vi "zad3 v0.0.2.vi"() -> ()   [LabVIEW 2017]
panel:
  in  "Interval (ms)":u32=500
  in  "stop":bool
  out "AIN3":dbl format="%.6f"
  out "AIN2":dbl format="%.6f"
  in  "FIO7":bool
  in  "FIO6":bool
  in  "DAC0":dbl format="%.4f"
  out "Error Message":string
  out "error out":errorcluster
  # "Outputs DAC0 and FIO6-FIO7.  Aquires AIN0-AIN3 and FIO4-FIO5.  This example\ndoes the proper pin configuration also.  Uses USB on the first found U3."
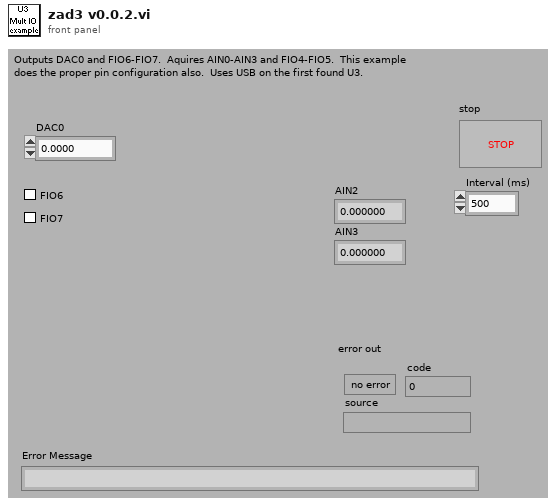
[diagram p1: front panel]
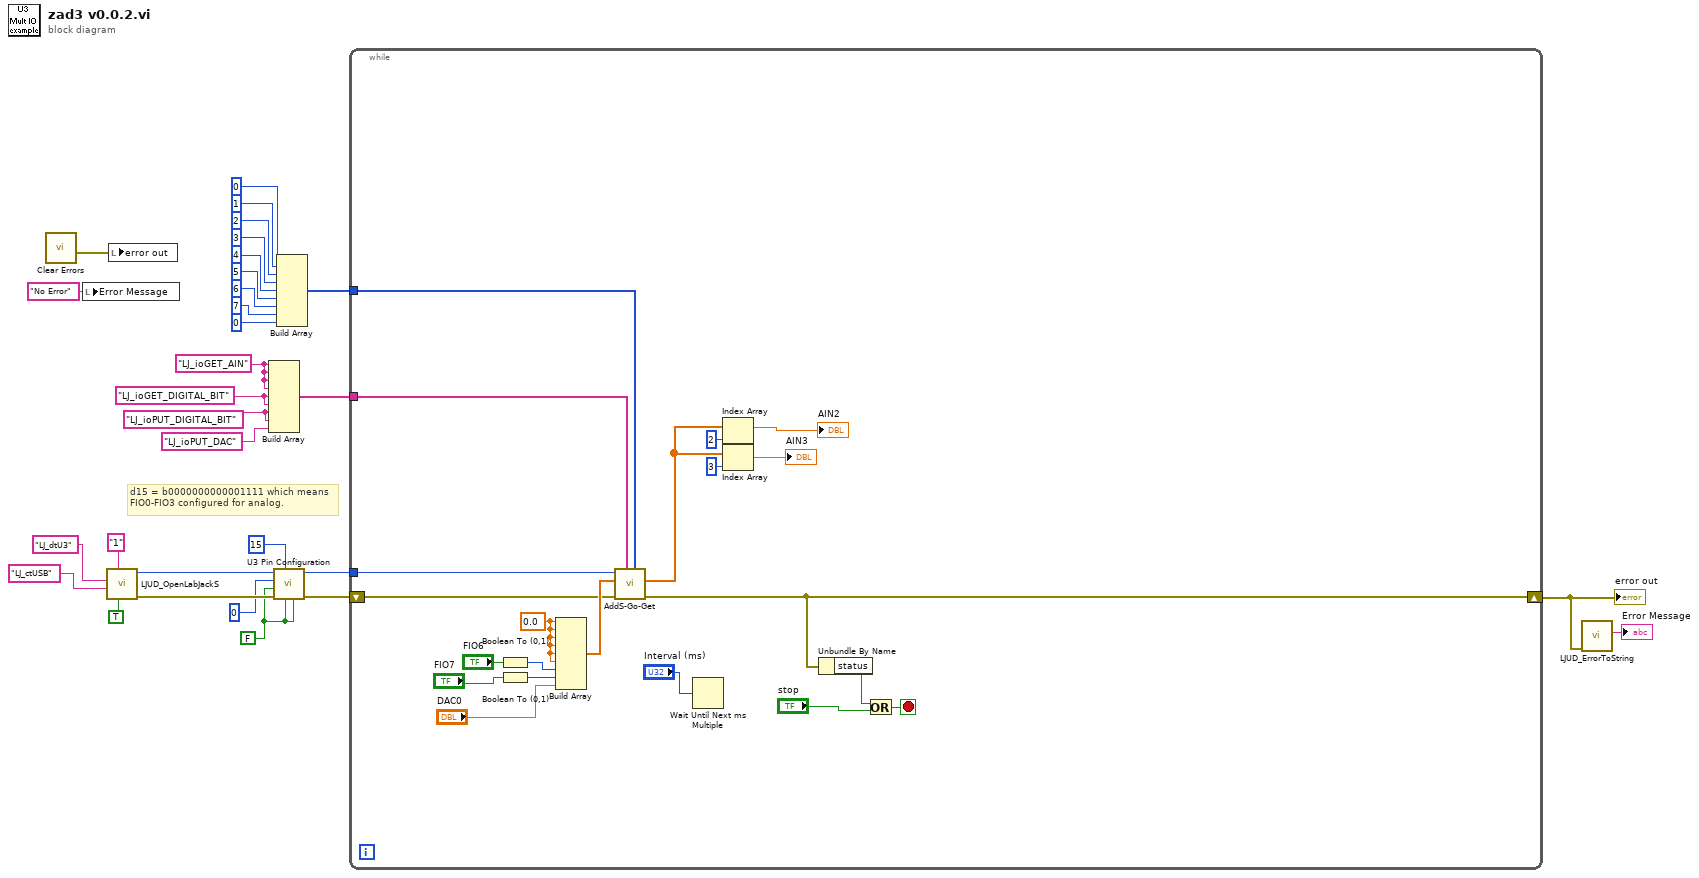
[diagram p0: block diagram]
diagram:
  w3 = FALSE ("Enable DAC1")
  w27 = "LJ_ioPUT_DIGITAL_BIT" ("IOType")
  w29 = "LJ_ioGET_AIN" ("IOType")
  w28 = "LJ_ioGET_DIGITAL_BIT" ("IOType")
  # "d15 = b0000000000001111 which means\nFIO0-FIO3 configured for analog."
  n1 = call <vilib>:"Clear Errors.vi"() -> ("error out"=w1:errorcluster)  [unwired: 6 in, 1 out]
  n2 = local write "Error Message"("No Error" ("Error Message")) -> ()
  n3 = call "LJUD_OpenLabJackS.vi"("FirstFound"=TRUE, "Address"="1", "ConnectionType"="LJ_ctUSB", "DeviceType"="LJ_dtU3") -> ("error out"=w8:errorcluster, "Handle"=w6:i32)  [unwired: 5 in, 1 out]
  n4 = local write "error out"(w1) -> ()
  n5 = Build Array(w29, w29, w29, w29, w28, w28, w27, w27, "LJ_ioPUT_DAC" ("IOType")) -> (w26:string[])
  n6 = call "U3 Pin Configuration.vi"("Enable Counter1"=w3, "Enable Counter0"=w3, "FIO/EIO Analog Enable"=15, "error in"=w8, "Enable DAC1"=w3, "Number of Timers Enabled"=u8 0, "Handle In"=w6) -> ("error out"=w9:errorcluster, "Handle Out"=w7:i32)  [unwired: 3 in]
  n7 = Build Array(0, 1, 2, 3, 4, 5, 6, 7, 0) -> (w25:i32[])
  n8 = while {
    shift-left: w9 -> [w33]
    shift-right: [w32] -> w10
    tunnel: w7 -> [w37]
    tunnel: w25 -> [w50]
    tunnel: w26 -> [w51]
    stop <- w36 stop-if-true
    w49 = 0.0 ("Input Element")
    n9 = Boolean To (0,1)(Boolean="FIO6") -> (0, 1=w48:i16)
    n10 = Boolean To (0,1)(Boolean="FIO7") -> (0, 1=w47:i16)
    n11 = Build Array(w49, w49, w49, w49, w49, w49, w48, w47, "DAC0") -> (w46:dbl[])
    n12 = call "AddS-Go-Get.vi"("Channels"=w50, "IOTypes"=w51, "error in"=w33, "Values Write"=w46, "Handle In"=w37) -> ("error out"=w32:errorcluster, "Values Read"=w43:dbl[])  [unwired: 4 in, 1 out]
    n13 = Wait Until Next ms Multiple(millisecond multiple="Interval (ms)") -> ()  [unwired: 1 out]
    n14 = Index Array(array=w43, index=2 ("Index")) -> (element=→"AIN2":dbl)
    n15 = Index Array(array=w43, index=3 ("Index")) -> (element=→"AIN3":dbl)
    n16 = Unbundle By Name(w32) -> ("status"=w34:bool)
    n17 = Or(x=w34, y="stop") -> (x .or. y?=w36:bool)
  }
  "error out" <- w10
  n18 = call "LJUD_ErrorToString.vi"("error in"=w10) -> ("String"=→"Error Message":string)  [unwired: 10 in]
